vi "GLIMPSE Globals.vi"() -> ()   [LabVIEW 2016]
uses:
  <vilib>/vision/Image Controls.llb/IMAQ Image.ctl
  Seq file v 1/Offset table.ctl
  Seq file v 1/Offset.ctl
  Seq file v 1/file number.ctl
  Image to Display event.ctt
  <vilib>/Utility/miscctls.llb/LVRectTypeDef.ctl
panel:
  in  "Display controller Presets":T1(array[cluster])=[{"Mem"=FALSE, "Black"=-32500.0, "White"=-25000.0, "Recall"=FALSE}]
  out "Display controller Window Bounds":T2={"Left"=0, "Top"=0, "Right"=100, "Bottom"=100}
  in  "Keep mage display controller in corner?":bool=TRUE
  out "Image controller display info":T4(array[cluster])
  in  "Current window Black/White Levels":cluster{ext, ext}(slide)={1.0, 65535.0} scale=0.0..255.0
  in  "Display image event":refnum<user-event>
  in  "Copy of Version string":string caption="Remember to make current value default!"
  in  "Serial Number for Image Buffers":i32
  out "Scratch Image 17":T3
  in  "Do One Fit Only?":bool=TRUE
  in  "IMAQ pixel depth":u32(ring) items=["8 bits", "16 bits", "Float", "Complex", "RGB", "HSL"]
  in  "VCR present?":bool
  out "Scratch Image 3":T3
  in  "Version string":string="GLIMPSE v. 54 (1/15)" caption="Remember to make current value default!"
  in  "Additional error information":string
  in  "RAID root path":path
  in  "Directory of last acquisition file accessed":path
  out "Region height":u16
  out "Region width":u16
  in  "File offsets":T5
  in  "Stop acquisition":bool
  out "Scratch Image 16":T3
  out "Scratch Image 2":T3
  out "Scratch Image 1":T3
  in  "Field mode":T8(ring)
  in  "Ring size":i32=100
  out "Ring buffer array":T3[](array[typedef])
  in  "Gain":dbl=1.0 format="%.2f"
  in  "Offset":dbl=5.0 format="%.2f"
  in  "time of 1st frame, \nsec since 1/1/04":dbl format="%.2f"
  in  "TTB Array (ms)":u32[](array[numeric])
  in  "Element 0 of TTB":u32
  in  "Hardware region being acquired":i32[](array[numeric])=[0, 0, 639, 479]
  in  "Sequence range":cluster{i16, i16}
  in  "Number of frames in sequence":u32
  # "IMAQ Hw Params"
  # "Properties of current sequence"
  # "Program Flags:"
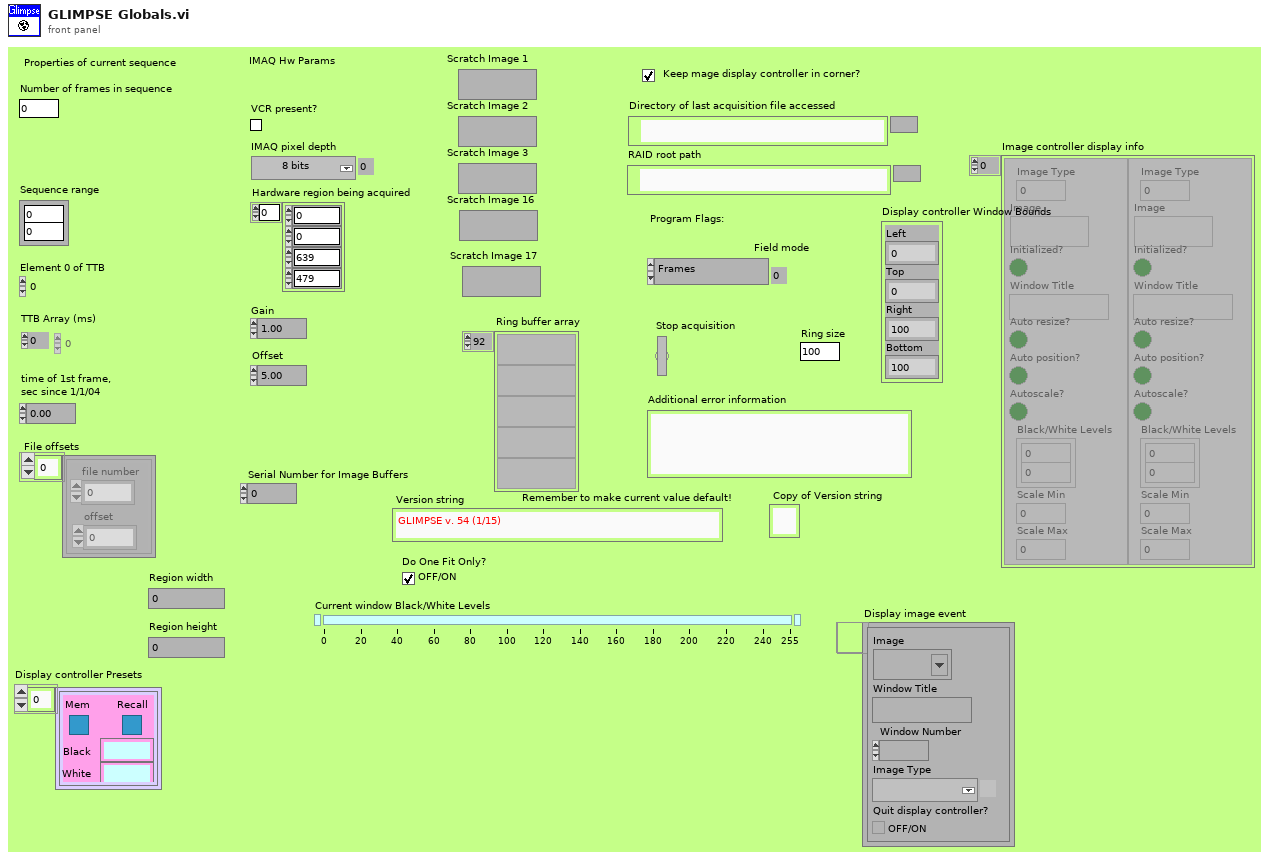
[diagram p1: front panel]
types:
  T1 = cluster{"Mem":bool, "Black":ext, "White":ext, "Recall":bool}[]
  T2 = typedef "LVRectTypeDef.ctl" = cluster{"Left":i16, "Top":i16, "Right":i16, "Bottom":i16}
  T3 = typedef "IMAQ Image.ctl" = refnum<image>
  T4 = cluster{"Image Type":u32, "Image":T3, "Initialized?":bool, "Window Title":string, "Auto resize?":bool, "Auto position?":bool, "Autoscale?":bool, "Black/White Levels":cluster{ext, ext}, "Scale Min":ext, "Scale Max":ext}[]
  T5 = typedef "Offset table.ctl" = cluster{"offset":T6, "file number":T7}[]
  T6 = typedef "Offset.ctl" = i32
  T7 = typedef "file number.ctl" = u8
  T8 = enum16{"Frames", "Fields, Odd 1st", "Fields, Even 1st", "Fields, Averaged"}
diagram:
